vi "round_to_decimal.vi"(1 "Value to Round":dbl=1.746, 2 "Number of Decimal\nPoints to Round to (4)":dbl=4.0) -> (0 "Rounded Value":dbl)   [LabVIEW 2017, in "sensor_translation.lvlib"]
uses:
  sensor_translation.lvlib
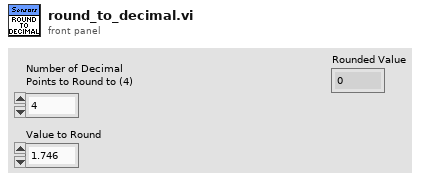
[diagram p1: front panel]
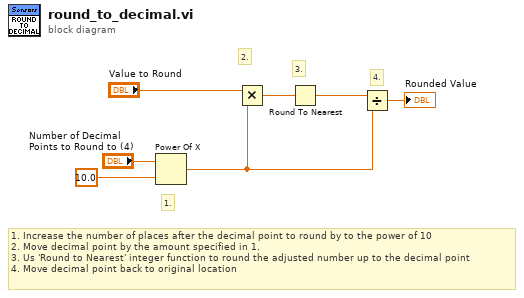
[diagram p0: block diagram]
diagram:
  # "3."
  # "1. Increase the number of places after the decimal point to round by to the power of 10\n2. Move decimal point by the amount specified in 1.\n3. Us 'Round to Nearest' integer function to round the adjusted number up to the decimal point\n4. Move decimal point back to original location"
  # "4."
  # "2."
  # "1."
  n1 = Power Of X(1:10.0 ("x"), 2:"Number of Decimal\nPoints to Round to (4)") -> (0:w2:dbl)
  n2 = Multiply(x="Value to Round", y=w2) -> (x*y=w4:dbl)
  n3 = Round To Nearest(number=w4) -> (nearest integer value=w3:dbl)
  n4 = Divide(x=w3, y=w2) -> (x/y=→"Rounded Value":dbl)
